vi "List-Item Name From ID and Name .vi"(7 "Separate Sign":string=".", 9 "Name":string, 10 "ID":i64=123456789, 11 "List":refnum<vi>) -> ()   [LabVIEW 2022 SP3]
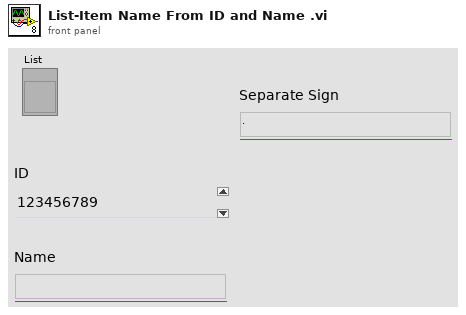
[diagram p1: front panel]
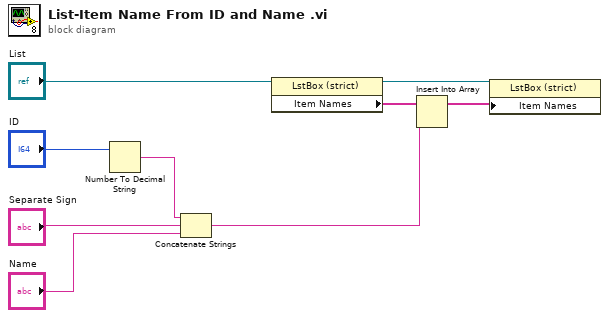
[diagram p0: block diagram]
diagram:
  n1 = Number To Decimal String(number="ID") -> (decimal integer string=w8:string)  [unwired: 1 in]
  n2 = Concatenate Strings(w8, "Separate Sign", "Name") -> (w1:string)
  n3 = property class="LstBox (strict)"(reference="List") -> (reference out=w3:refnum<vi>, "Item Names"=w4:string[])  [unwired: 1 in, 1 out]
  n4 = Insert Into Array(array=w4, new element=w1) -> (w2:string[])  [unwired: 1 in]
  n5 = property class="LstBox (strict)"(reference=w3, "Item Names"=w2) -> ()  [unwired: 1 in, 2 out]
